vi "Read CPU Load Data.vi"(8 "error in (no error)":errorcluster, 11 "Sequence Directory In":path) -> (0 "error out":errorcluster, 2 "XY Graph Data":cluster{dbl[], dbl[]}, 3 "Sequence Directory Out":path)   [LabVIEW 2015]
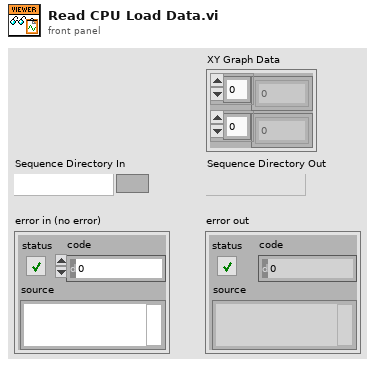
[diagram p1: front panel]
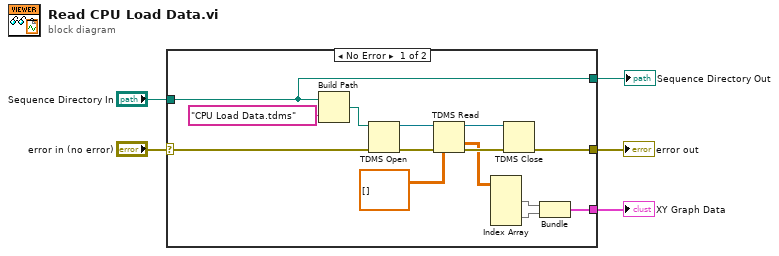
[diagram p0: block diagram]
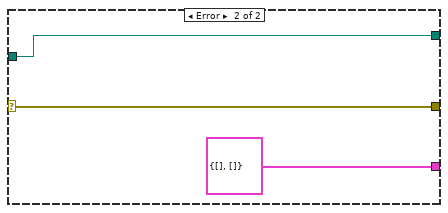
[diagram p2: hidden frame]
diagram:
  n1 = case shown="No Error" "error in (no error)" {
    selector: "error in (no error)" -> [w10 w22]
    tunnel: "Sequence Directory In" -> [w6 w20]
    tunnel: [w8 w22] -> w3
    tunnel: [w7 cluster{dbl[], dbl[]} {[], []}] -> w2
    tunnel: [w6 w20] -> w1
    frame No Error {
      n2 = Build Path(base path=w6, name or relative path="CPU Load Data.tdms") -> (appended path=w9:path)
      n3 = TDMS Open(8:w10, 11:w9) -> (0:w17:errorcluster, 3:w18:refnum<k34>)  [unwired: 5 in]
      n4 = TDMS Read(0:w18, 11:w17, 12:dbl[][] []) -> (4:w15:refnum<k34>, 10:w13:dbl[][], 15:w14:errorcluster)  [unwired: 5 in, 3 out]
      n5 = Index Array(array=w13) -> (element #1=w12:dbl[], element #2=w11:dbl[])  [unwired: 4 in]
      n6 = TDMS Close(8:w14, 11:w15) -> (0:w8:errorcluster)  [unwired: 1 out]
      n7 = Bundle(w12, w11) -> (w7:cluster{dbl[], dbl[]})  [unwired: 1 in]
    }
    frame Error {
    }
  }
  "error out" <- w3
  "XY Graph Data" <- w2
  "Sequence Directory Out" <- w1
